vi "RTS Wago Points.vi"(7 "Point Data":T2[](array[typedef]), 8 "Error In":errorcluster, 9 "Wago Data":string[](array[string]), 11 "Input Save Array":T1[](array[typedef])) -> (0 "Error Out":errorcluster, 3 "Output Save Array":T1[](array[typedef]))   [LabVIEW 2019]
uses:
  Washer DOE/Type Definitions/DOE Data Save Modifier.ctl
  Type Definitions/RTS Point File.ctl
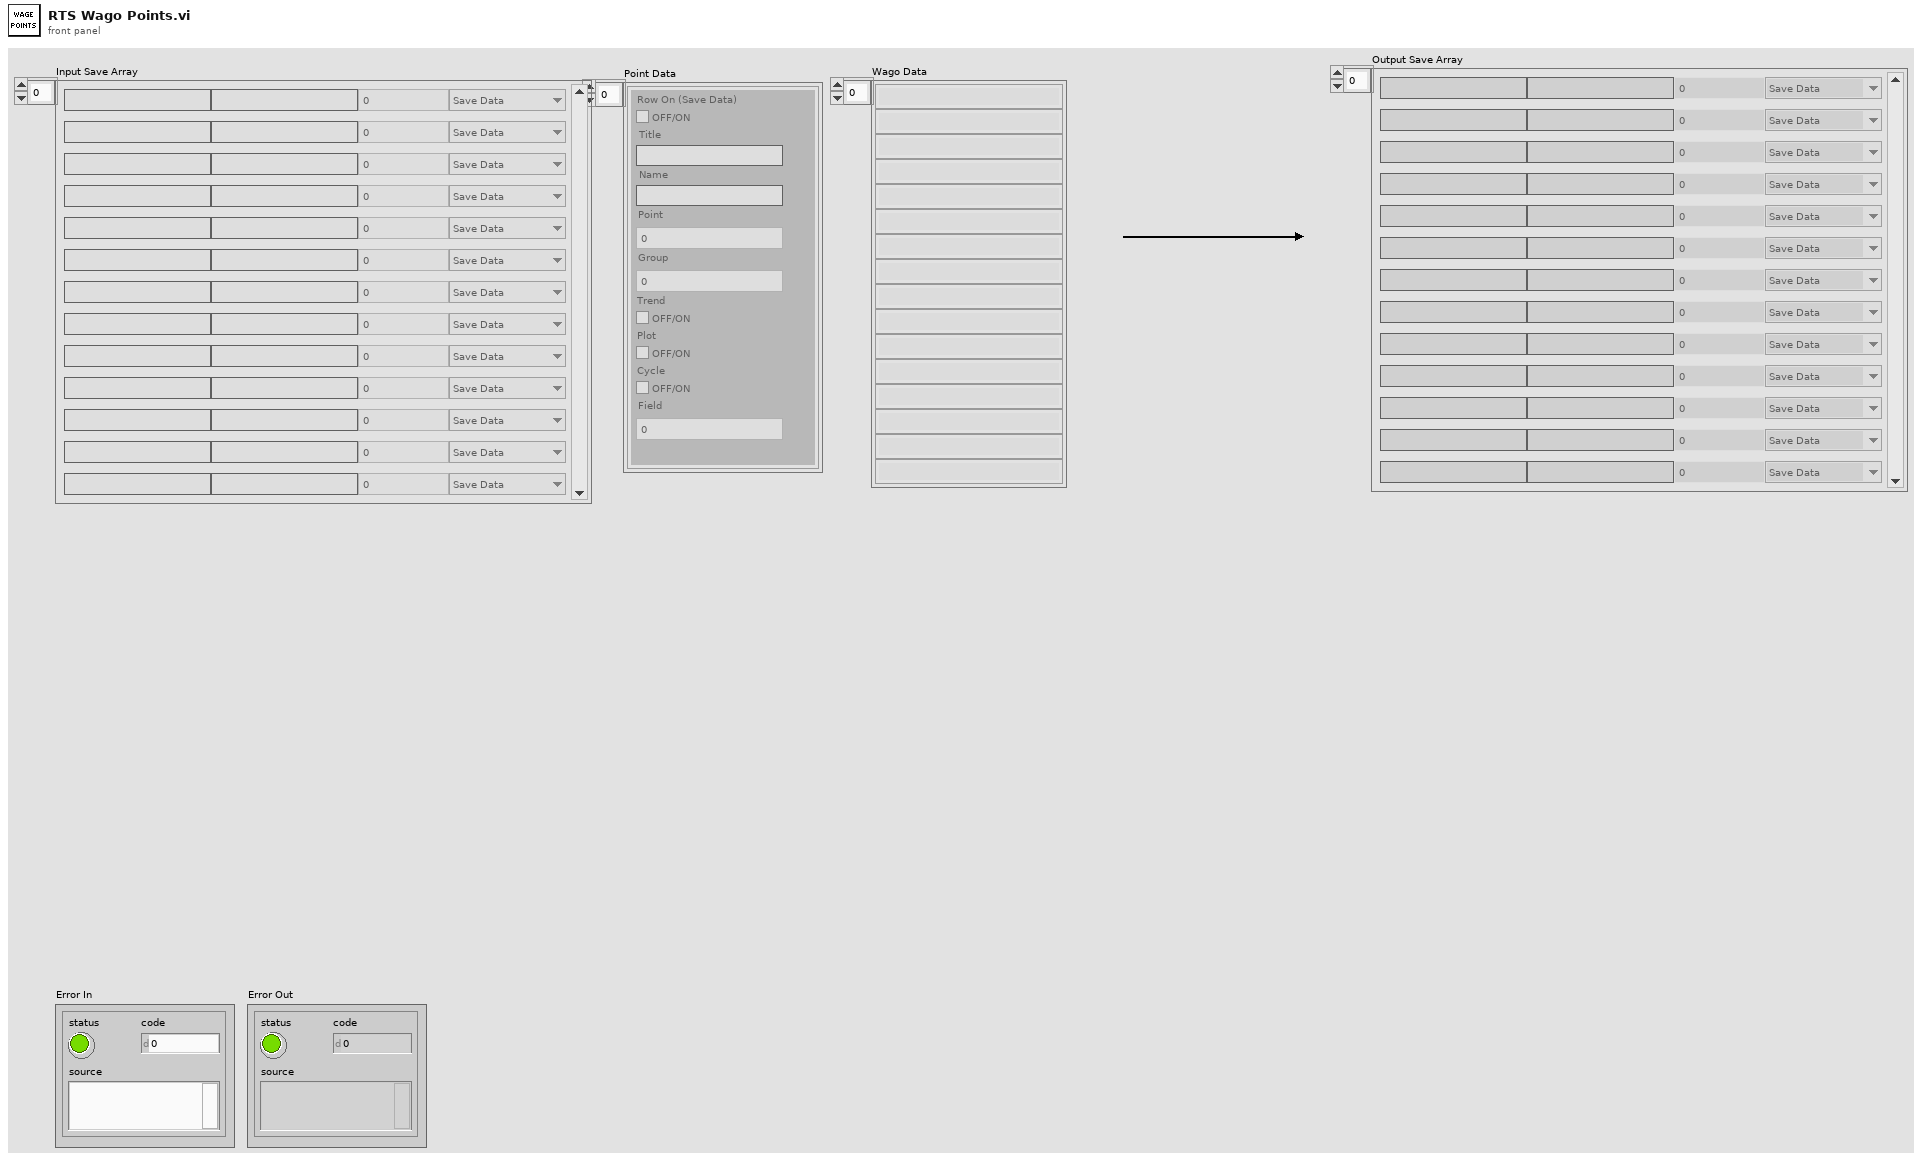
[diagram p1: front panel]
types:
  T1 = typedef "DOE Data Save Modifier.ctl" = cluster{"Name":string, "Title":string, "Save Status":enum16{"Save Data", "Don't Save Data"}, "Group":u8, "Field":u8}
  T2 = typedef "RTS Point File.ctl" = cluster{"Title":string, "Name":string, "Point":u8, "Plot":bool, "Trend":bool, "Cycle":bool, "Field":u8, "Row On (Save Data)":bool, "Group":u8}
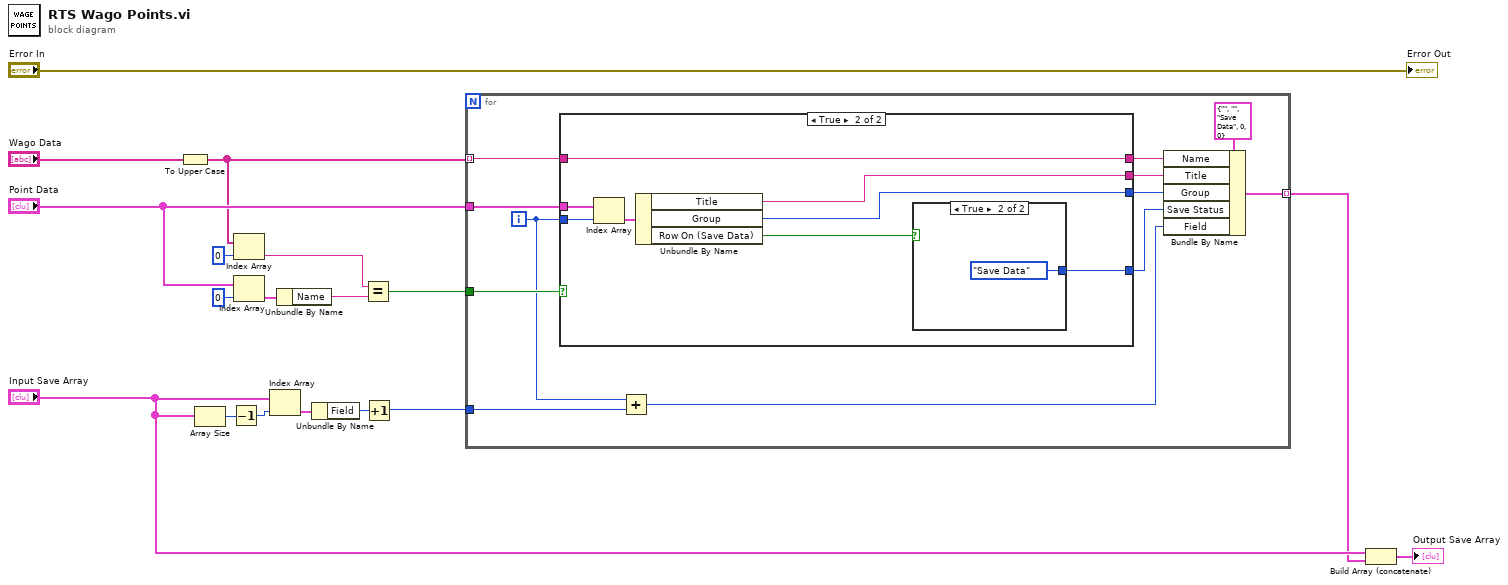
[diagram p0: block diagram]
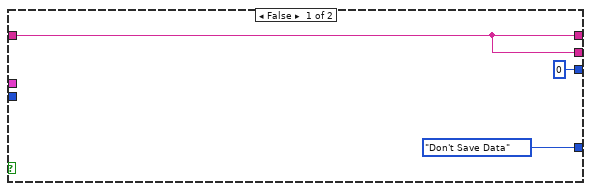
[diagram p2: hidden frame]
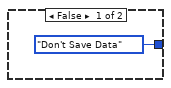
[diagram p3: hidden frame]
diagram:
  n1 = To Upper Case(1:"Wago Data") -> (0:w1:string[])
  n2 = Array Size(array="Input Save Array") -> (size(s)=w15:i32)
  n3 = Decrement(x=w15) -> (x-1=w16:i32)
  n4 = Index Array(array=w1, index=0) -> (element=w2:string)
  n5 = Index Array(array="Point Data", index=0) -> (element=w10:T2)
  n6 = Index Array(array="Input Save Array", index=w16) -> (element=w14:T1)
  n7 = Unbundle By Name(w10) -> ("Name"=w11:string)
  n8 = Unbundle By Name(w14) -> ("Field"=w17:u8)
  n9 = Equal?(x=w2, y=w11) -> (x = y?=w6:bool)
  n10 = Increment(x=w17) -> (x+1=w5:u8)
  n11 = for {
    tunnel: "Point Data" -> [w26]
    tunnel: [w27] -> w12 mode=indexing
    tunnel: w1 -> [w24] mode=indexing
    tunnel: w6 -> [w25]
    tunnel: w5 -> [w20]
    i -> [w21]
    n12 = case shown="True" w25 {
      tunnel: [w33 w41] -> w29
      tunnel: [u8 0 ("Group") w40] -> w28
      tunnel: w26 -> [_ w39]
      tunnel: w21 -> [_ w38]
      tunnel: w24 -> [w33 w36]
      tunnel: [w33 w36] -> w23
      tunnel: [enum16{"Save Data", "Don't Save Data"}."Don't Save Data" ("Save Status") w35] -> w22
      frame False {
      }
      frame True {
        n13 = Index Array(array=w39, index=w38) -> (element=w37:T2)
        n14 = Unbundle By Name(w37) -> ("Title"=w41:string, "Group"=w40:u8, "Row On (Save Data)"=w34:bool)
        n15 = case shown="True" w34 {
          tunnel: [enum16{"Save Data", "Don't Save Data"}."Don't Save Data" ("Save Status") enum16{"Save Data", "Don't Save Data"}."Save Data" ("Save Status")] -> w35
          frame False {
          }
          frame True {
          }
        }
      }
    }
    n16 = Add(x=w21, y=w20) -> (x+y=w19:i32)
    n17 = Bundle By Name(cluster=T1 {"Name"="", "Title"="", "Save Status"=enum."Save Data", "Group"=0, "Field"=0} ("Cluster"), "Name"=w23, "Title"=w29, "Group"=w28, "Save Status"=w22, "Field"=w19) -> (w27:T1)
  }
  n18 = Build Array (concatenate)("Input Save Array", w12) -> (→"Output Save Array":T1[])
  "Error Out" <- "Error In"
